vi "Or_60_Seconds.vi"(11 "10MHz?":bool) -> (3 "10MHz?_60s":bool, 5 "array":bool[](array[boolean]))   [LabVIEW 2018]
doc: "If 10 MHz reference drops out for even one sample, report the minute as an error."
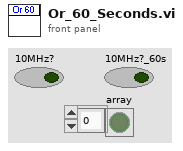
[diagram p1: front panel]
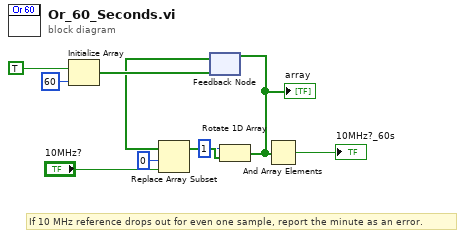
[diagram p0: block diagram]
diagram:
  # "If 10 MHz reference drops out for even one sample, report the minute as an error."
  n1 = Initialize Array(TRUE, 60 ("dimension size")) -> (w5:bool[])
  n2 = feedback #1(w5) -> (w3:bool[])
  n3 = Replace Array Subset(array=w3, new element="10MHz?", index=0) -> (w9:bool[])
  n4 = Rotate 1D Array(1:w9, 2:1 ("n")) -> (0:w4:bool[])
  "array" <- w4
  n5 = feedback-in #1(w4) -> ()
  n6 = And Array Elements(Boolean array=w4) -> (logical AND=→"10MHz?_60s":bool)
